vi "Player Info.vi"(8 "Victory Speech":string="Resistance is Futile", 9 "Name":string="Net", 11 "Net in":refnum<class "Net.lvclass">) -> (3 "Net out":refnum<class "Net.lvclass">)   [LabVIEW 2015, in "Net.lvclass"]
uses:
  Net.lvclass
  Square/Square.lvclass
panel:
  # "Set default values for these two string controls"
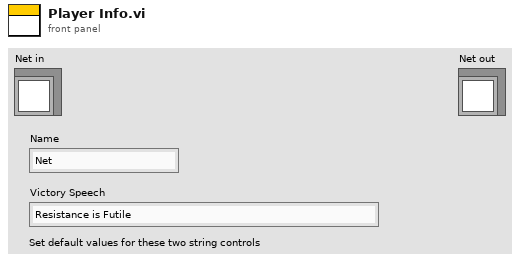
[diagram p1: front panel]
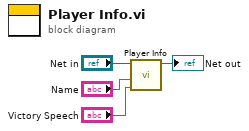
[diagram p0: block diagram]
diagram:
  n1 = call-parent "Player Info.vi"("Victory Speech"="Victory Speech", "Name"="Name", "Square in"="Net in") -> ("Square out"=→"Net out":refnum<class "Net.lvclass">)  [unwired: 8 in]
